vi "Do Read.vi"(8 "error in (no error)":errorcluster, 9 "Timeout ms":i32, 10 "Count":i32, 11 "WebsocketStream in":refnum<class "WebsocketStream.lvclass">) -> (0 "error out":errorcluster, 1 "Remaining  Timeout":i32, 2 "Data":string, 3 "WebsocketStream out":refnum<class "WebsocketStream.lvclass">)   [LabVIEW 2020, in "Stream-Websocket.lvlib" / "WebsocketStream.lvclass"]
uses:
  WebsocketStream.lvclass
  WebsocketStream.lvclass/WebsocketStream.ctl
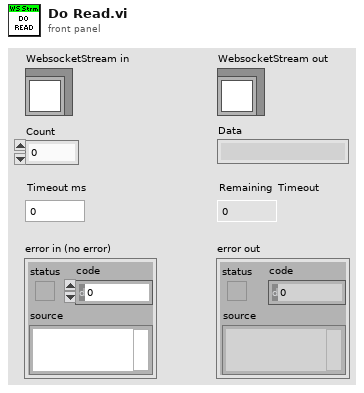
[diagram p1: front panel]
types:
  T1 = enum16{"Standard", "Buffered", "CRLF", "Immediate"}
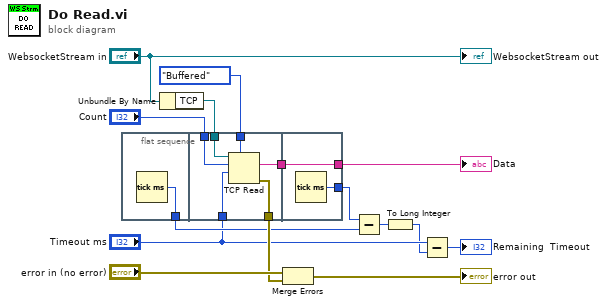
[diagram p0: block diagram]
diagram:
  n1 = flat-sequence {
    tunnel: [w16] -> w6
    tunnel: T1."Buffered" ("mode (standard)") -> [w22]
    tunnel: [w21] -> w11
    tunnel: [w20] -> w9
    tunnel: w8 -> [w19]
    tunnel: "Count" -> [w18]
    tunnel: "Timeout ms" -> [w17]
    tunnel: [w24] -> w12
    tunnel: w11 -> [w24]
    tunnel: [w23] -> w5
    frame #0 {
      n2 = Tick Count (ms)() -> (millisecond timer value=w16:u32)
    }
    frame #1 {
      n3 = TCP Read(connection ID=w19, bytes to read=w18, 7:w22, 9:w17) -> (data out=w21:string, error out=w20:errorcluster)  [unwired: 1 in, 1 out]
    }
    frame #2 {
      n4 = Tick Count (ms)() -> (millisecond timer value=w23:u32)
    }
  }
  n5 = Unbundle By Name("WebsocketStream in") -> ("TCP"=w8:refnum<k5>)
  n6 = Merge Errors("error in (no error)", w9) -> (→"error out":errorcluster)
  n7 = Subtract(x=w5, y=w6) -> (x-y=w3:u32)
  n8 = To Long Integer(number=w3) -> (32bit integer=w1:i32)
  n9 = Subtract(x="Timeout ms", y=w1) -> (x-y=→"Remaining  Timeout":i32)
  "WebsocketStream out" <- "WebsocketStream in"
  "Data" <- w12
